vi "TableFinalizerRole.vi"(6 "Tactic index in":i32, 7 "first call":bool, 8 "error in (no error)":errorcluster, 10 "Game in":refnum<class "Game.lvclass">, 11 "TableFinalizerRole in":refnum<class "TableFinalizerRole.lvclass">) -> (0 "error out":errorcluster, 1 "tactic index":i32, 2 "Robot out":refnum<class "Robot.lvclass">, 3 "TableFinalizerRole out":refnum<class "TableFinalizerRole.lvclass">)   [LabVIEW 2021, in "TableFinalizerRole.lvclass"]
uses:
  TableFinalizerRole.lvclass
  Game_class/Game.lvclass
  Robot_class/Robot.lvclass
  D:/RoboIme/horie/SSL_AI/Role_class/Role.lvclass
  Role_class/Role.lvclass/Role.ctl
  TableFinalizerRole.lvclass/TableFinalizerRole.ctl
  KickToPassReceiverTactic_class/KickToPassReceiverTacticStates.ctl
  KickToPassReceiverTactic_class/KickToPassReceiverTactic.lvclass/KickToPassReceiverTactic.ctl
  Tacticbook_class/Tacticbook.lvclass/Tacticbook.ctl
  ShootTactic_class/States.ctl
  ShootTactic_class/ShootTactic.lvclass/ShootTactic.ctl
  KickToPassReceiverTactic_class/Read States.vi
  Tacticbook_class/Read WaitPassTactic.vi
  Tacticbook_class/Write WaitPassTactic.vi
  Tacticbook_class/Read ShootTactic.vi
  ShootTactic_class/Read States.vi
  Tacticbook_class/Write ShootTactic.vi
  Role_class/Read Tacticbook.vi
  Read number_of_tactics.vi
  Role_class/Write Tacticbook.vi
  Role_class/Write tactic_index.vi
  Role_class/Read RobotRef.vi
  Tacticbook_class/Tacticbook.lvclass
  KickToPassReceiverTactic_class/KickToPassReceiverTactic.lvclass
  WaitPassTactic_class/WaitPassTactic.lvclass
  ShootTactic_class/ShootTactic.lvclass
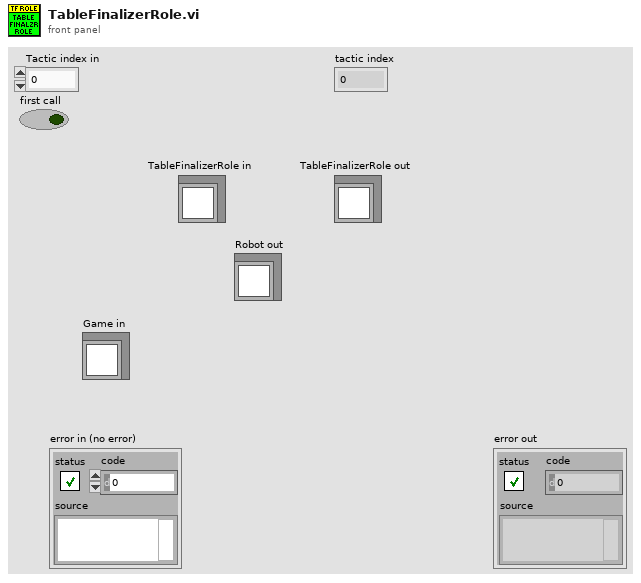
[diagram p1: front panel]
types:
  T1 = typedef "KickToPassReceiverTacticStates.ctl" = enum16{"Halt", "GoToReceiveTable", "KickToPassReceiver", "WaitPass", "Exit"}
  T2 = typedef "ShootTactic.lvclass/States.ctl" = enum16{"BallInGoalieArea", "Exit", "KickToGoal", "StealBall"}
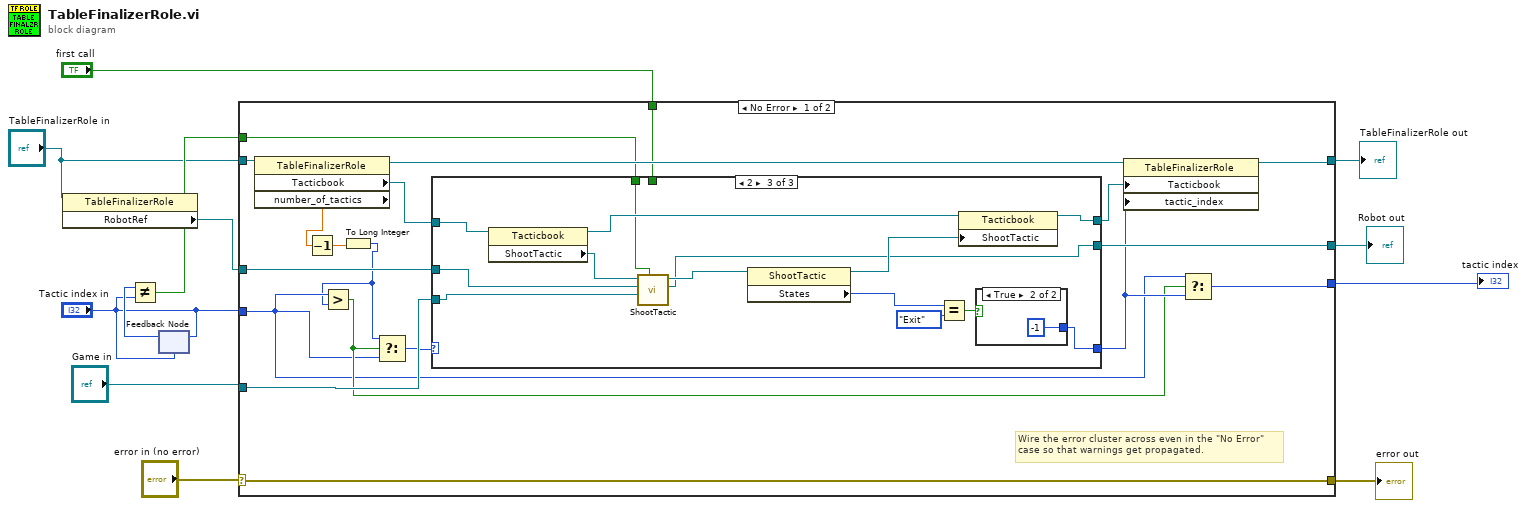
[diagram p0: block diagram]
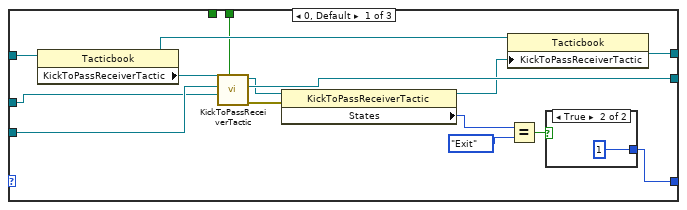
[diagram p2: hidden frame]
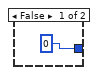
[diagram p3: hidden frame]
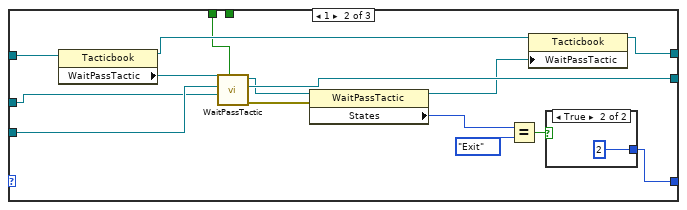
[diagram p4: hidden frame]
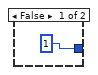
[diagram p5: hidden frame]
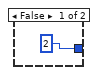
[diagram p6: hidden frame]
diagram:
  n1 = property class="TableFinalizerRole"(reference="TableFinalizerRole in") -> ("RobotRef"=w10:refnum<class "Robot.lvclass">)  [unwired: 1 in, 2 out]
  n2 = feedback #1("Tactic index in") -> (w6:i32)
  n3 = Not Equal?(x=w6, y="Tactic index in") -> (x != y?=w4:bool)
  n4 = feedback-in #1("Tactic index in") -> ()
  n5 = case shown="No Error" "error in (no error)" {
    selector: "error in (no error)" -> [w31 w84]
    tunnel: [w31 w84] -> w11
    tunnel: [w29 w83] -> w1
    tunnel: "TableFinalizerRole in" -> [w30 w83]
    tunnel: w10 -> [w26 w82]
    tunnel: [w25 w82] -> w3
    tunnel: "Game in" -> [w23 _]
    tunnel: [w21 _] -> w9
    tunnel: "Tactic index in" -> [w18 _]
    tunnel: "first call" -> [w16 _]
    tunnel: w4 -> [w13 _]
    frame No Error {
      # "Wire the error cluster across even in the \"No Error\"\ncase so that warnings get propagated."
      n6 = property class="TableFinalizerRole"(reference=w30) -> (reference out=w28:refnum<class "TableFinalizerRole.lvclass">, "Tacticbook"=w27:refnum<class "Tacticbook.lvclass">, "number_of_tactics"=w17:dbl)  [unwired: 1 in, 1 out]
      n7 = Decrement(x=w17) -> (x-1=w15:dbl)
      n8 = To Long Integer(number=w15) -> (32bit integer=w14:i32)
      n9 = Greater?(x=w18, y=w14) -> (0:w19:bool)
      n10 = Select(t=w14, s=w19, f=w18) -> (s? t:f=w20:i32)
      n11 = case shown="2" w20 {
        tunnel: [w34 w51 w68] -> w22
        tunnel: w27 -> [w46 w63 w77]
        tunnel: w26 -> [w37 w54 w70]
        tunnel: [w45 w62 w71] -> w25
        tunnel: [w41 w58 w75] -> w24
        tunnel: w23 -> [w38 w55 w69]
        tunnel: w16 -> [w33 _ _]
        tunnel: w13 -> [_ w50 w66]
        frame 0, Default {
          n12 = property class="Tacticbook"(reference=w46) -> (reference out=w43:refnum<class "Tacticbook.lvclass">, "KickToPassReceiverTactic"=w40:refnum<class "KickToPassReceiverTactic.lvclass">)  [unwired: 1 in, 1 out]
          n13 = call "KickToPassReceiverTactic.vi"("first call"=w33, "Robot"=w37, "Game in"=w38, "KickToPassReceiverTactic in"=w40) -> ("error out"=w44:errorcluster, "Robot out"=w45:refnum<class "Robot.lvclass">, "KickToPassReceiverTactic out"=w39:refnum<class "KickToPassReceiverTactic.lvclass">)  [unwired: 5 in]
          n14 = property class="KickToPassReceiverTactic"(reference=w39, error in=w44) -> (reference out=w42:refnum<class "KickToPassReceiverTactic.lvclass">, "States"=w35:T1)  [unwired: 1 out]
          n15 = property class="Tacticbook"(reference=w43, "KickToPassReceiverTactic"=w42) -> (reference out=w41:refnum<class "Tacticbook.lvclass">)  [unwired: 1 in, 1 out]
          n16 = Equal?(x=w35, y=KickToPassReceiverTacticStates."Exit") -> (x = y?=w36:bool)
          n17 = case shown="True" w36 {
            tunnel: [0 1] -> w34
            frame False {
            }
            frame True {
            }
          }
        }
        frame 1 {
          n18 = property class="Tacticbook"(reference=w63) -> (reference out=w60:refnum<class "Tacticbook.lvclass">, "WaitPassTactic"=w57:refnum<class "WaitPassTactic.lvclass">)  [unwired: 1 in, 1 out]
          n19 = call-dynamic "WaitPassTactic.vi"("first call"=w50, "Robot"=w54, "Game in"=w55, "WaitPassTactic in"=w57) -> ("error out"=w61:errorcluster, "Robot out"=w62:refnum<class "Robot.lvclass">, "WaitPassTactic out"=w56:refnum<class "WaitPassTactic.lvclass">)  [unwired: 5 in]
          n20 = property class="WaitPassTactic"(reference=w56, error in=w61) -> (reference out=w59:refnum<class "WaitPassTactic.lvclass">, "States"=w52:enum16{"State 0", "State 1", "State 2", "Exit"})  [unwired: 1 out]
          n21 = Equal?(x=w52, y=enum16{"State 0", "State 1", "State 2", "Exit"}."Exit") -> (x = y?=w53:bool)
          n22 = property class="Tacticbook"(reference=w60, "WaitPassTactic"=w59) -> (reference out=w58:refnum<class "Tacticbook.lvclass">)  [unwired: 1 in, 1 out]
          n23 = case shown="True" w53 {
            tunnel: [1 2] -> w51
            frame False {
            }
            frame True {
            }
          }
        }
        frame 2 {
          n24 = property class="Tacticbook"(reference=w77) -> (reference out=w76:refnum<class "Tacticbook.lvclass">, "ShootTactic"=w73:refnum<class "ShootTactic.lvclass">)  [unwired: 1 in, 1 out]
          n25 = call "ShootTactic.vi"("firstCall?"=w66, "Game in"=w69, "Robot"=w70, "ShootTactic in"=w73) -> ("Robot out"=w71:refnum<class "Robot.lvclass">, "ShootTactic out"=w72:refnum<class "ShootTactic.lvclass">)  [unwired: 4 in, 2 out]
          n26 = property class="ShootTactic"(reference=w72) -> (reference out=w74:refnum<class "ShootTactic.lvclass">, "States"=w78:T2)  [unwired: 1 in, 1 out]
          n27 = Equal?(x=w78, y=States."Exit") -> (x = y?=w79:bool)
          n28 = property class="Tacticbook"(reference=w76, "ShootTactic"=w74) -> (reference out=w75:refnum<class "Tacticbook.lvclass">)  [unwired: 1 in, 1 out]
          n29 = case shown="True" w79 {
            tunnel: [2 -1] -> w68
            frame False {
            }
            frame True {
            }
          }
        }
      }
      n30 = property class="TableFinalizerRole"(reference=w28, "Tacticbook"=w24, "tactic_index"=w22) -> (reference out=w29:refnum<class "TableFinalizerRole.lvclass">)  [unwired: 1 in, 1 out]
      n31 = Select(t=w18, s=w19, f=w22) -> (s? t:f=w21:i32)
    }
    frame Error {
    }
  }
  "error out" <- w11
  "tactic index" <- w9
  "Robot out" <- w3
  "TableFinalizerRole out" <- w1
